vi "Periodic Tasks.vi"(8 "error in":errorcluster) -> ()   [LabVIEW 2017]
doc: "This VI runs in parallel to other tasks. It can contain as many user-defined periodic loops as you need. These can carry out PID or other sorts of timed response."
uses:
  <vilib>/Rock Robotics/WPI/Utilities/WPI_GetSetVariantRefNum.vi
  <vilib>/Rock Robotics/Network Tables/NT Read Number.vi
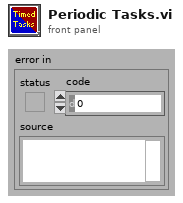
[diagram p1: front panel]
types:
  T1 = typedef "WPI_JoystickDevRef.ctl" = cluster{"Device":T2}
  T2 = typedef "WPI_JoystickDeviceEnum.ctl" = enum16{"USB 0", "USB 1", "USB 2", "USB 3", "USB 4", "USB 5"}
  T3 = typedef "WPI_RobotDriveDevRef.ctl" = cluster{"DevStatus":errorcluster, "Motors[]":T4[], "Square Inputs":bool, "Max Output":dbl}
  T4 = typedef "WPI_MotorControlDeviceRef.ctl" = cluster{"DeviceStatus":errorcluster, "Type":T5, "PWM":cluster{"PWM Channel":T6, "DeadBand":T7}, "CAN":cluster{"Device Number":u8, "SetOutput VI Ref":variant, "GetOutput VI Ref":variant, "Enable VI Ref":variant, "Disable VI Ref":variant, "Data":variant}, "Invert":bool, "DIO PWM":cluster{"PWM \"Enable\" Channel":T6, "DIOChannel":T8, "PWM Rate":dbl}}
  T5 = typedef "WPI_MotorControlType.ctl" = enum16{"PWM", "CAN", "DIO PWM"}
  T6 = typedef "FPGA_DIOPWMChannel.ctl" = enum8{"PWM 0", "PWM 1", "PWM 2", "PWM 3", "PWM 4", "PWM 5", "PWM 6", "PWM 7", "PWM 8", "PWM 9", "PWM MXP 0", "PWM MXP 1", "PWM MXP 2", "PWM MXP 3", "PWM MXP 4", "PWM MXP 5", "PWM MXP 6", "PWM MXP 7", "PWM MXP 8", "PWM MXP 9", "Invalid"}
  T7 = typedef "WPI_PWMDeadband.ctl" = cluster{"Name":string, "maxPositivePwm":i32, "minPositivePwm":i32, "centerPwm":i32, "maxNegativePwm":i32, "minNegativePwm":i32, "angularRange":u16}
  T8 = typedef "FPGA_DIOChannel.ctl" = enum8{"DIO 0", "DIO 1", "DIO 2", "DIO 3", "DIO 4", "DIO 5", "DIO 6", "DIO 7", "DIO 8", "DIO 9", "DIO MXP 0", "DIO MXP 1", "DIO MXP 2", "DIO MXP 3", "DIO MXP 4", "DIO MXP 5", "DIO MXP 6", "DIO MXP 7", "DIO MXP 8", "DIO MXP 9", "DIO MXP 10", "DIO MXP 11", "DIO MXP 12", "DIO MXP 13", "DIO MXP 14", "DIO MXP 15", "SPI Port CS1", "SPI Port CS2", "SPI Port CS3", "SPI Port MISO", "SPI Port MOSI", "Invalid"}
  T9 = cluster{"JoystickDevRef":T1, "RobotDriveDevRef":T3}
  T10 = cluster{"offsetAngle H":dbl, "offsetAngle V":dbl, "area":dbl, "skew":dbl, "target":dbl}
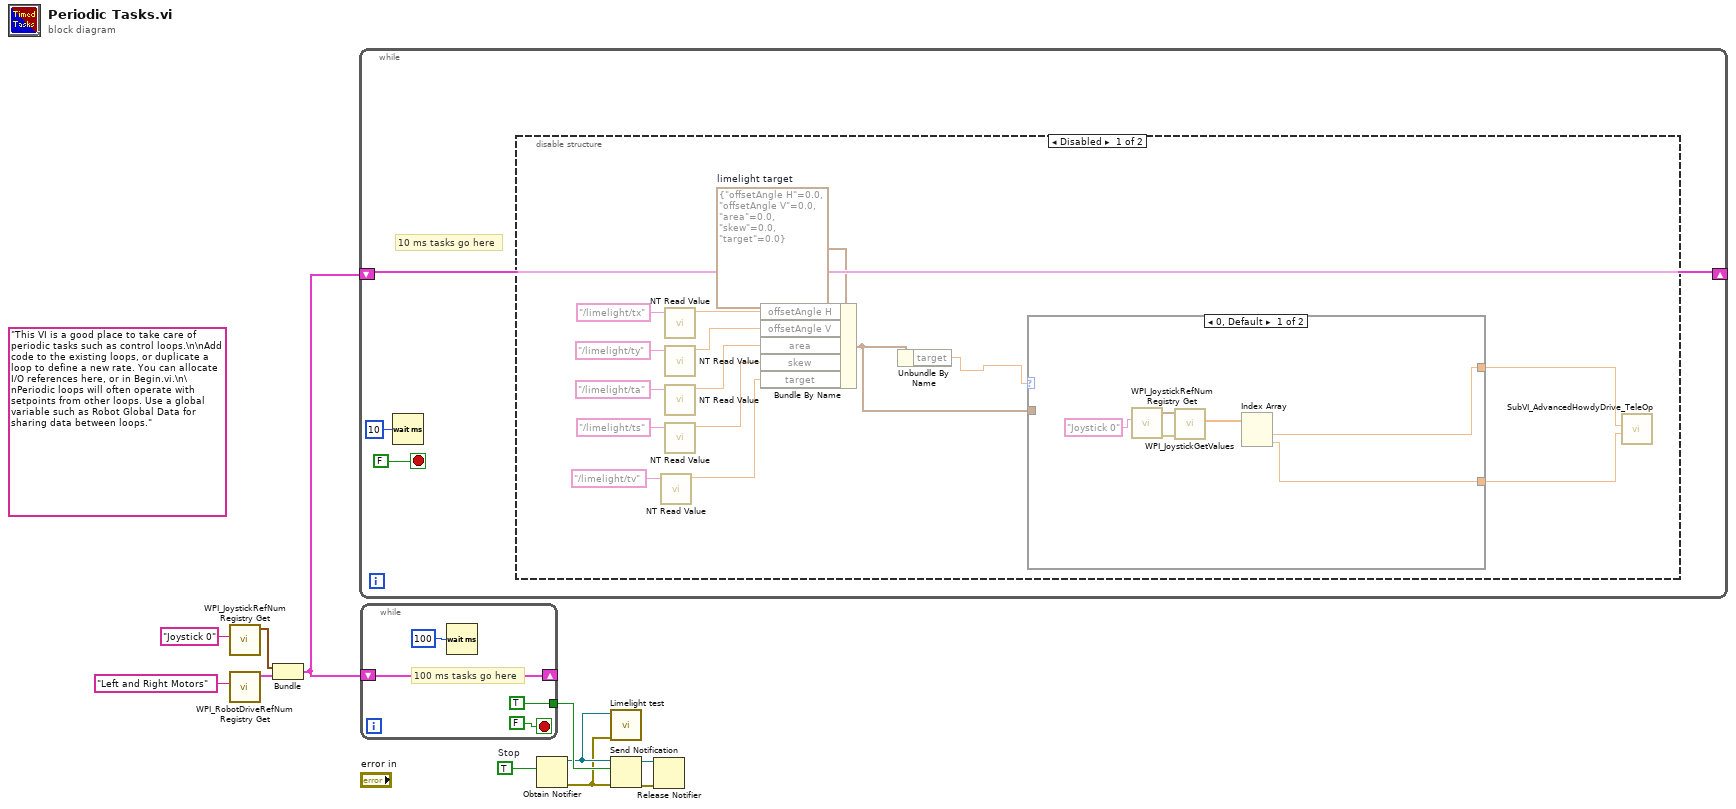
[diagram p0: block diagram]
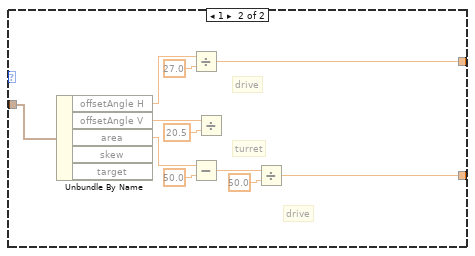
[diagram p2: hidden frame]
diagram:
  w6 = TRUE  # Stop
  (unwired) "This VI is a good place to take care of periodic tasks such as control loops.\n\nAdd code to the existing loops, or duplicate a loop to define a new rate. You can allocate I/O references here, or in Begin.vi.\n\nPeriodic loops will often operate with setpoints from other loops. Use a global variable such as Robot Global Data for sharing data between loops."
  n1 = call <vilib>:"WPI_JoystickRefNum Registry Get.vi"("refnum name"="Joystick 0") -> ("JoystickDevRef"=w9:T1)  [unwired: 1 in, 9 out]
  n2 = call <vilib>:"WPI_RobotDriveRefNum Registry Get.vi"("refnum name"="Left and Right Motors") -> ("RobotDriveDevRef"=w8:T3)  [unwired: 1 in, 9 out]
  n3 = Bundle("JoystickDevRef"=w9, "RobotDriveDevRef"=w8) -> (w7:T9)  [unwired: 1 out]
  n4 = while {
    shift-right: [w12] -> _
    shift-left: w7 -> [w12]
    stop <- FALSE stop-if-true
    # "10 ms tasks go here"
    n5 = Wait (ms)(milliseconds to wait=u32 10) -> ()  [unwired: 1 out]
    n6 = disable-structure shown="Disabled" {
      frame Disabled {
        w25 = T10 {"offsetAngle H"=0.0, "offsetAngle V"=0.0, "area"=0.0, "skew"=0.0, "target"=0.0}  # limelight target
        n7 = call-poly <vilib>:"NT Read Value.vi"("Name"="/limelight/tv") -> ("Numeric"=w19:dbl)  [unwired: 9 in, 1 out]
        n8 = call-poly <vilib>:"NT Read Value.vi"("Name"="/limelight/tx") -> ("Numeric"=w24:dbl)  [unwired: 9 in, 1 out]
        n9 = call-poly <vilib>:"NT Read Value.vi"("Name"="/limelight/ty") -> ("Numeric"=w23:dbl)  [unwired: 9 in, 1 out]
        n10 = call-poly <vilib>:"NT Read Value.vi"("Name"="/limelight/ta") -> ("Numeric"=w22:dbl)  [unwired: 9 in, 1 out]
        n11 = call-poly <vilib>:"NT Read Value.vi"("Name"="/limelight/ts") -> ("Numeric"=w21:dbl)  [unwired: 9 in, 1 out]
        n12 = Bundle By Name(cluster=w25, "offsetAngle H"=w24, "offsetAngle V"=w23, "area"=w22, "skew"=w21, "target"=w19) -> (w17:T10)
        n13 = Unbundle By Name(w17) -> ("target"=w18:dbl)
        n14 = case shown="0, Default" w18 {
          tunnel: w17 -> [_ w46]
          tunnel: [w31 w37] -> w16
          tunnel: [w32 w36] -> w15
          frame 0, Default {
            n15 = call <vilib>:"WPI_JoystickRefNum Registry Get.vi"("refnum name"="Joystick 0") -> ("error out"=w35:errorcluster, "JoystickDevRef"=w30:T1)  [unwired: 9 in]
            n16 = call <vilib>:"WPI_JoystickGetValues.vi"("error in (no error)"=w35, "JoystickDevRef"=w30) -> ("Axes"=w33:dbl[])  [unwired: 5 in, 4 out]
            n17 = Index Array(array=w33) -> (element #1=w32:dbl, element #2=w31:dbl)  [unwired: 2 in]
          }
          frame 1 {
            # "drive"
            # "drive"
            # "turret"
            n18 = Unbundle By Name(w46) -> ("offsetAngle H"=w45:dbl, "offsetAngle V"=w43:dbl, "area"=w41:dbl)  [unwired: 2 out]
            n19 = Divide(x=w45, y=27.0) -> (x/y=w36:dbl)
            n20 = Subtract(x=w41, y=50.0) -> (x-y=w39:dbl)
            n21 = Divide(x=w43, y=20.5) -> ()  [unwired: 1 out]
            n22 = Divide(x=w39, y=50.0) -> (x/y=w37:dbl)
          }
        }
        n23 = call "SubVI_AdvancedHowdyDrive_TeleOp.vi"("Y axis value"=w16, "X axis value"=w15) -> ()  [unwired: 8 in, 2 out]
      }
      frame Enabled {
      }
    }
  }
  n24 = while {
    shift-right: [w48] -> _
    shift-left: w7 -> [w48]
    tunnel: [TRUE] -> w5
    stop <- FALSE stop-if-true
    # "100 ms tasks go here"
    n25 = Wait (ms)(milliseconds to wait=u32 100) -> ()  [unwired: 1 out]
  }
  n26 = Obtain Notifier(notification data type=w6) -> (notifier out=w4:refnum<notifier>, error out=w3:errorcluster)  [unwired: 3 in, 1 out]
  n27 = call "Limelight test.vi"("error in (no error)"=w3, "Notifier In"=w4) -> ()  [unwired: 9 in, 1 out]
  n28 = Send Notification(notification=w5, notifier=w4, error in (no error)=w3) -> (notifier out=w2:refnum<notifier>, error out=w1:errorcluster)
  n29 = Release Notifier(notifier=w2, error in (no error)=w1) -> ()  [unwired: 1 in, 3 out]
